vi "Init.vi"(7 "Cluster":T1, 8 "error in (no error)":errorcluster, 9 "Init or Array":bool, 10 "Array":dbl[](array[numeric]), 11 "All Channels in":refnum<class "All Channels Out.lvclass">) -> (0 "error out":errorcluster, 3 "All Channels out":refnum<class "All Channels Out.lvclass">)   [LabVIEW 2018, in "All Channels Out.lvclass"]
uses:
  All Channels Out.lvclass
  Scaling/Scaling.lvclass
  All Channels Out.lvclass/All Channels Out.ctl
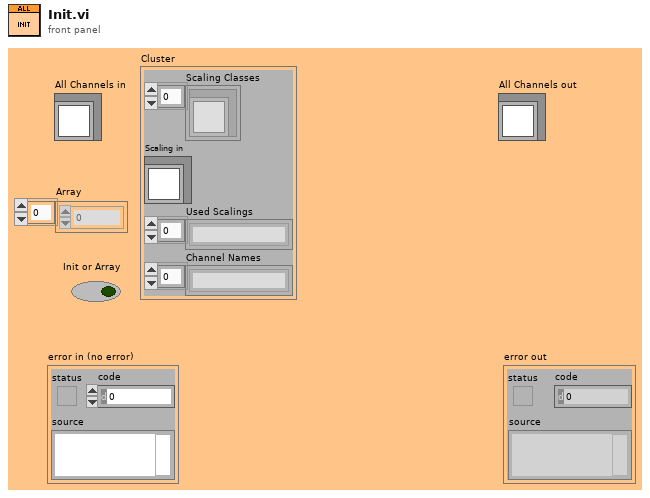
[diagram p1: front panel]
types:
  T1 = cluster{"Scaling Classes":refnum<class "Scaling.lvclass">[], "Scaling in":refnum<class "Scaling.lvclass">, "Used Scalings":string[], "Channel Names":string[]}
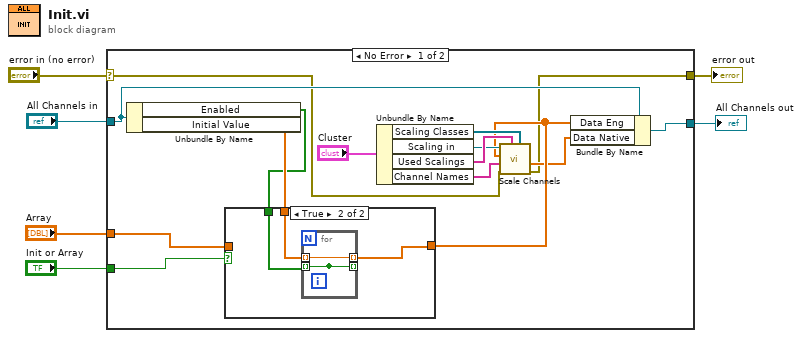
[diagram p0: block diagram]
diagram:
  n1 = case shown="No Error" "error in (no error)" {
    selector: "error in (no error)" -> [w8 w32]
    tunnel: [w7 w32] -> w5
    tunnel: [w21 w33] -> w4
    tunnel: "All Channels in" -> [w20 w33]
    tunnel: "Init or Array" -> [w19 _]
    tunnel: "Array" -> [w17 _]
    frame No Error {
      n2 = Unbundle By Name(w20) -> ("Enabled"=w16:bool[], "Initial Value"=w18:dbl[])
      n3 = case shown="True" w19 {
        tunnel: w18 -> [_ w28]
        tunnel: [w22 w27] -> w10
        tunnel: w17 -> [w23 _]
        tunnel: w16 -> [w24 w29]
        frame False {
          n4 = for {
            tunnel: [w25] -> w22 mode=indexing if=w26
            tunnel: w24 -> [w26] mode=indexing
            tunnel: [w26] -> _ mode=indexing
            tunnel: w23 -> [w25] mode=indexing
          }
        }
        frame True {
          n5 = for {
            tunnel: [w30] -> w27 mode=indexing if=w31
            tunnel: w29 -> [w31] mode=indexing
            tunnel: [w31] -> _ mode=indexing
            tunnel: w28 -> [w30] mode=indexing
          }
        }
      }
      n6 = Unbundle By Name("Cluster") -> ("Scaling Classes"=w12:refnum<class "Scaling.lvclass">[], "Scaling in"=w13:refnum<class "Scaling.lvclass">, "Used Scalings"=w14:string[], "Channel Names"=w15:string[])
      n7 = call "Scale Channels.vi"("Scaling Classes"=w12, "Used Scalings"=w14, "error in (no error)"=w8, "Channel Names"=w15, "Values In"=w10, "Scaling in"=w13) -> ("error out"=w7:errorcluster, "Values Out"=w9:dbl[])  [unwired: 3 in, 1 out]
      n8 = Bundle By Name(cluster=w20, "Data Eng"=w10, "Data Native"=w9) -> (w21:refnum<class "All Channels Out.lvclass">)
    }
    frame Error {
    }
  }
  "error out" <- w5
  "All Channels out" <- w4
